vi "基础15.vi"() -> ()   [LabVIEW 2014]
panel:
  out "字符串 2":string
  in  "字符串":string
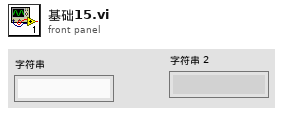
[diagram p1: front panel]
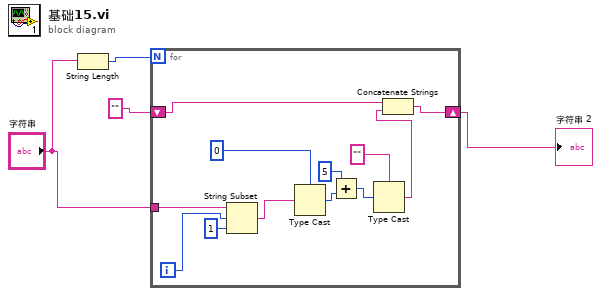
[diagram p0: block diagram]
diagram:
  n1 = String Length(string="字符串") -> (length=w4:i32)
  n2 = for {
    N: w4 -> [_]
    tunnel: "字符串" -> [w16]
    shift-right: [w5] -> w1
    shift-left: "" -> [w7]
    i -> [w14]
    n3 = String Subset(string=w16, offset (0)=w14, length (rest)=1 ("长度（剩余）")) -> (substring=w12:string)
    n4 = Type Cast(type=u8 0, x=w12) -> (*(type *) &x=w9:u8)
    n5 = Add(x=u8 5, y=w9) -> (x+y=w8:u8)
    n6 = Type Cast(type="", x=w8) -> (*(type *) &x=w6:string)
    n7 = Concatenate Strings(w7, w6) -> (w5:string)
  }
  "字符串 2" <- w1
